vi "CHD_DRIVE_MODULE_OPEN.vi"(3 "Module Index":i32, 5 "Drive PWM Channel":T2, 6 "DistancePerCount":dbl=1.0, 8 "Reverse":bool, 10 "Drive B Channel":T1, 11 "Drive A channel":T1) -> ()   [LabVIEW 2019]
uses:
  <vilib>/Rock Robotics/WPI/MotorControl/WPI_MotorControlOpen SPARK.vi
  <vilib>/Rock Robotics/WPI/Counter/WPI_CounterDigitalInputToDigitalSource.vi
  <vilib>/Rock Robotics/WPI/SafetyOutput/WPI_SafetyOutputConfigMenu.ctl
  <vilib>/Rock Robotics/WPI/Encoder/WPI_EncoderType.ctl
  <vilib>/Rock Robotics/SystemInterfaces/DIO/FPGA_DIOChannel.ctl
  <vilib>/Rock Robotics/SystemInterfaces/DIO/FPGA_DIOPWMChannel.ctl
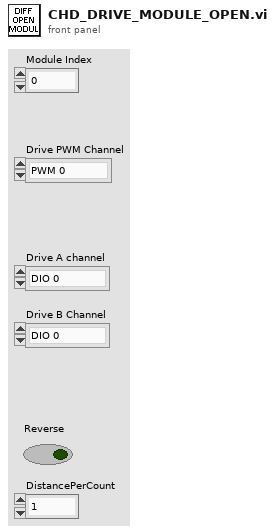
[diagram p1: front panel]
types:
  T1 = typedef "FPGA_DIOChannel.ctl" = enum8{"DIO 0", "DIO 1", "DIO 2", "DIO 3", "DIO 4", "DIO 5", "DIO 6", "DIO 7", "DIO 8", "DIO 9", "DIO MXP 0", "DIO MXP 1", "DIO MXP 2", "DIO MXP 3", "DIO MXP 4", "DIO MXP 5", "DIO MXP 6", "DIO MXP 7", "DIO MXP 8", "DIO MXP 9", "DIO MXP 10", "DIO MXP 11", "DIO MXP 12", "DIO MXP 13", "DIO MXP 14", "DIO MXP 15", "SPI Port CS1", "SPI Port CS2", "SPI Port CS3", "SPI Port MISO", "SPI Port MOSI", "Invalid"}
  T2 = typedef "FPGA_DIOPWMChannel.ctl" = enum8{"PWM 0", "PWM 1", "PWM 2", "PWM 3", "PWM 4", "PWM 5", "PWM 6", "PWM 7", "PWM 8", "PWM 9", "PWM MXP 0", "PWM MXP 1", "PWM MXP 2", "PWM MXP 3", "PWM MXP 4", "PWM MXP 5", "PWM MXP 6", "PWM MXP 7", "PWM MXP 8", "PWM MXP 9", "Invalid"}
  T3 = typedef "WPI_EncoderType.ctl" = enum16{"1x", "2x", "4x"}
  T4 = typedef "WPI_SafetyOutputConfigMenu.ctl" = enum16{"Enable", "Disable"}
  T5 = typedef "WPI_MotorControlDeviceRef.ctl" = cluster{"DeviceStatus":errorcluster, "Type":T6, "PWM":cluster{"PWM Channel":T2, "DeadBand":T7}, "CAN":cluster{"Device Number":u8, "SetOutput VI Ref":variant, "GetOutput VI Ref":variant, "Enable VI Ref":variant, "Disable VI Ref":variant, "Data":variant}, "Invert":bool, "DIO PWM":cluster{"PWM \"Enable\" Channel":T2, "DIOChannel":T1, "PWM Rate":dbl}}
  T6 = typedef "WPI_MotorControlType.ctl" = enum16{"PWM", "CAN", "DIO PWM"}
  T7 = typedef "WPI_PWMDeadband.ctl" = cluster{"Name":string, "maxPositivePwm":i32, "minPositivePwm":i32, "centerPwm":i32, "maxNegativePwm":i32, "minNegativePwm":i32, "angularRange":u16}
  T8 = typedef "WPI_DigitalInputDevRef.ctl" = cluster{"DevStatus":errorcluster, "DIO Channel":T1}
  T9 = typedef "FPGA_CounterEncoderSourceConvertionLVSourceType.ctl" = cluster{"DevStatus":errorcluster, "AnalogTriggerMode?":bool, "DigitalMode":cluster{"DIO Channel":T10}, "AnalogTriggerMode":cluster{"AnalogTriggerIndex":T11, "OutputType":T12}}
  T10 = typedef "FPGA_DIODigitalSourceChannel.ctl" = enum8{"DIO 0", "DIO 1", "DIO 2", "DIO 3", "DIO 4", "DIO 5", "DIO 6", "DIO 7", "DIO 8", "DIO 9", "DIO MXP 0", "DIO MXP 1", "DIO MXP 2", "DIO MXP 3", "DIO MXP 4", "DIO MXP 5", "DIO MXP 6", "DIO MXP 7", "DIO MXP 8", "DIO MXP 9", "DIO MXP 10", "DIO MXP 11", "DIO MXP 12", "DIO MXP 13", "DIO MXP 14", "DIO MXP 15", "SPI Port CS1", "SPI Port CS2", "SPI Port CS3", "SPI Port MISO", "SPI Port MOSI", "Disabled"}
  T11 = typedef "FPGA_AnalogTriggerIndex.ctl" = enum8{"Trig 0", "Trig 1", "Trig 2", "Trig 3", "Trig 4", "Trig 5", "Trig 6", "Trig 7", "Invalid"}
  T12 = typedef "FPGA_AnalogTriggerOutType.ctl" = enum16{"InWindow", "TriggerState", "Rising", "Falling"}
  T13 = typedef "WPI_EncoderDevRef.ctl" = cluster{"DevStatus":errorcluster, "EncoderIndex":T14, "CounterIndex":T15, "DistancePerCount":dbl, "Decoding Type":T3}
  T14 = typedef "FPGA_EncoderIdx.ctl" = enum8{"Enc 0", "Enc 1", "Enc 2", "Enc 3", "Enc 4", "Enc 5", "Enc 6", "Enc 7", "Invalid"}
  T15 = typedef "FPGA_CounterCtrSystemIndex.ctl" = enum8{"Ctr 0", "Ctr 1", "Ctr 2", "Ctr 3", "Ctr 4", "Ctr 5", "Ctr 6", "Ctr 7", "Invalid"}
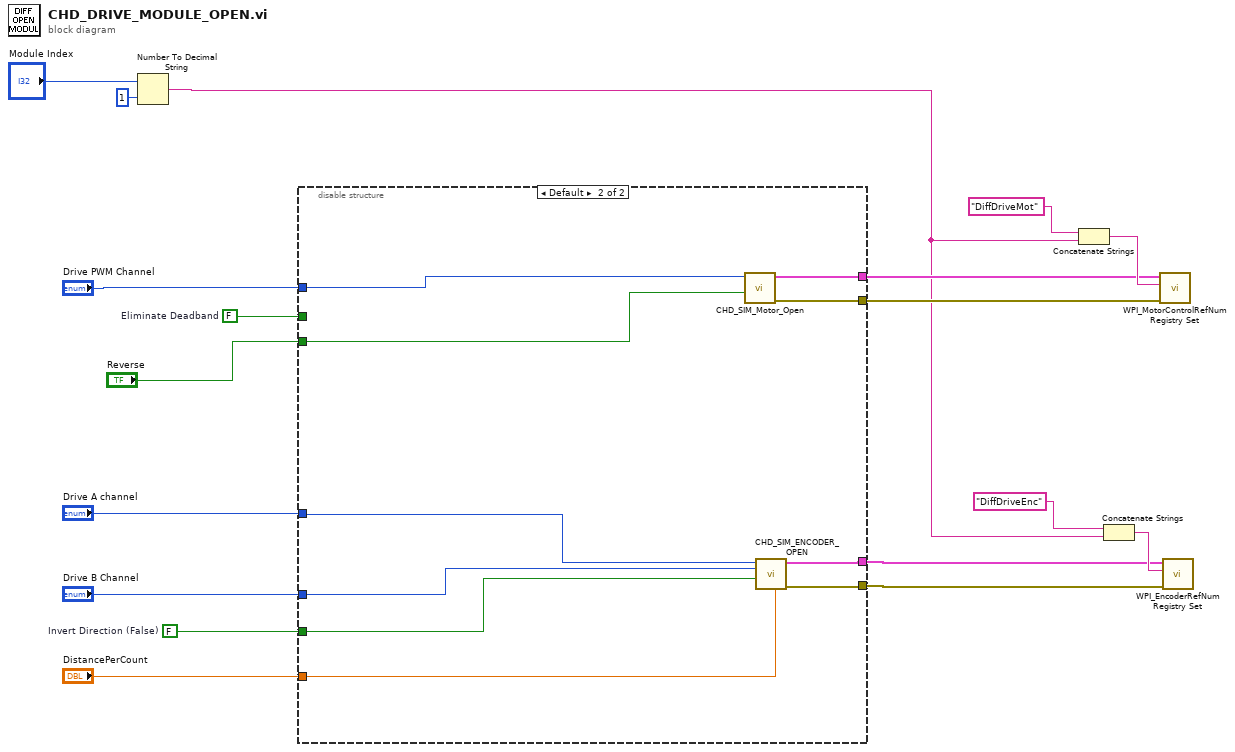
[diagram p0: block diagram]
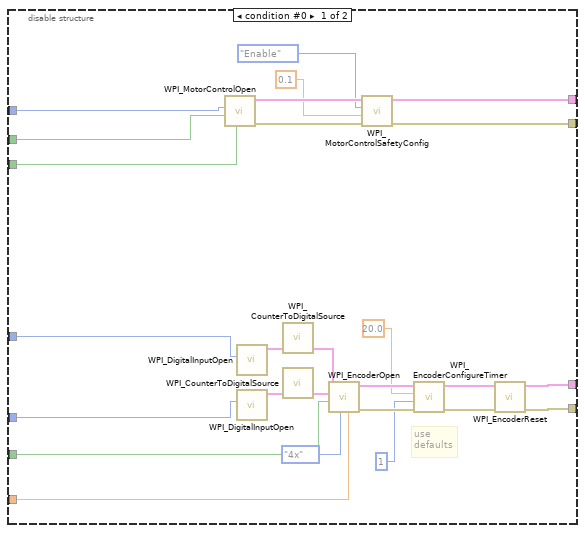
[diagram p2: hidden frame]
diagram:
  w3 = FALSE  # Eliminate Deadband
  w4 = FALSE  # Invert Direction (False)
  n1 = Number To Decimal String(number="Module Index", width (-)=i16 1) -> (decimal integer string=w1:string)
  n2 = disable-structure shown="Default" {
    disable-tunnel: "Drive B Channel" -> [w32 w51]
    disable-tunnel: "Drive A channel" -> [w31 w52]
    disable-tunnel: "DistancePerCount" -> [w30 w49]
    disable-tunnel: "Drive PWM Channel" -> [w28 w48]
    disable-tunnel: [w27 w46] -> w8
    disable-tunnel: [w26 w47] -> w7
    disable-tunnel: [w23 w53] -> w6
    disable-tunnel: [w22 w54] -> w5
    disable-tunnel: w4 -> [w21 w50]
    disable-tunnel: "Reverse" -> [w20 w45]
    disable-tunnel: w3 -> [w19 _]
    frame condition #0 {
      # "use\ndefaults"
      n3 = call-poly <vilib>:"WPI_MotorControlOpen.vi"("Invert"=w20, "Eliminate Deadband"=w19, "PWM Channel"=w28) -> ("error out"=w39:errorcluster, "MotorControlDeviceRef"=w40:T5)  [unwired: 7 in]
      n4 = call <vilib>:"WPI_DigitalInputOpen.vi"("DIO Channel"=w31) -> ("DigitalInputDevRef"=w42:T8)  [unwired: 1 in, 9 out]
      n5 = call <vilib>:"WPI_DigitalInputOpen.vi"("DIO Channel"=w32) -> ("DigitalInputDevRef"=w43:T8)  [unwired: 1 in, 9 out]
      n6 = call-poly <vilib>:"WPI_CounterToDigitalSource.vi"("DigitalInputDevRef"=w42) -> ("Digital Source"=w41:T9)  [unwired: 6 out]
      n7 = call-poly <vilib>:"WPI_CounterToDigitalSource.vi"("DigitalInputDevRef"=w43) -> ("Digital Source"=w44:T9)  [unwired: 6 out]
      n8 = call <vilib>:"WPI_EncoderOpen.vi"("DistancePerCount"=w30, "Decoding Type"=WPI_EncoderType."4x", "Invert Direction (False)"=w21, "BSource"=w44, "ASource"=w41) -> ("error out"=w37:errorcluster, "EncoderDevRef"=w38:T13)  [unwired: 3 in, 2 out]
      n9 = call <vilib>:"WPI_MotorControlSafetyConfig.vi"("error in (no error)"=w39, "timeout (s)"=0.1, "mode"=WPI_SafetyOutputConfigMenu."Enable", "MotorControlDevRef"=w40) -> ("error out"=w27:errorcluster, "MotorControlDevRef"=w26:T5)  [unwired: 6 in]
      n10 = call <vilib>:"WPI_EncoderConfigureTimer.vi"("error in (no error)"=w37, "Number Samples to Average"=u8 1, "Minimum Rate"=20.0, "EncoderDevRef"=w38) -> ("error out"=w25:errorcluster, "EncoderDevRef"=w24:T13)  [unwired: 6 in]
      n11 = call <vilib>:"WPI_EncoderReset.vi"("error in (no error)"=w25, "EncoderDevRef"=w24) -> ("error out"=w23:errorcluster, "EncoderDevRef"=w22:T13)  [unwired: 8 in]
    }
    frame condition #1 (active) {
      n12 = call "CHD_SIM_Motor_Open.vi"("Invert"=w45, "PWM Channel"=w48) -> ("error out"=w46:errorcluster, "Motor Device Reference"=w47:T5)  [unwired: 8 in]
      n13 = call "CHD_SIM_ENCODER_OPEN.vi"("DistancePerCount"=w49, "Invert"=w50, "DIO Channel B"=w51, "DIO Channel  A"=w52) -> ("error out"=w53:errorcluster, "SwerveDriveEnc"=w54:T13)  [unwired: 6 in]
    }
  }
  n14 = Concatenate Strings("DiffDriveMot" ("refnum name"), w1) -> (w9:string)
  n15 = Concatenate Strings("DiffDriveEnc" ("refnum name"), w1) -> (w10:string)
  n16 = call <vilib>:"WPI_MotorControlRefNum Registry Set.vi"("error in (no error)"=w8, "refnum name"=w9, "MotorControlDevRef"=w7) -> ()  [unwired: 7 in, 2 out]
  n17 = call <vilib>:"WPI_EncoderRefNum Registry Set.vi"("error in (no error)"=w6, "refnum name"=w10, "EncoderDevRef"=w5) -> ()  [unwired: 7 in, 2 out]
